vi "Send Packets.vi"(8 "error in (no error)":errorcluster, 9 "Delay before packets, sec":dbl=0.1 format="%#_13g", 10 "SG Power, dBm":dbl, 11 "IVI Refnum in":refnum<k15>) -> (0 "error out":errorcluster, 3 "IVI Refnum out":refnum<k15>)   [LabVIEW 2025, in "Nordic nRF52 DK DTM Test.lvlib"]
uses:
  Nordic nRF52 DK DTM Test.lvlib
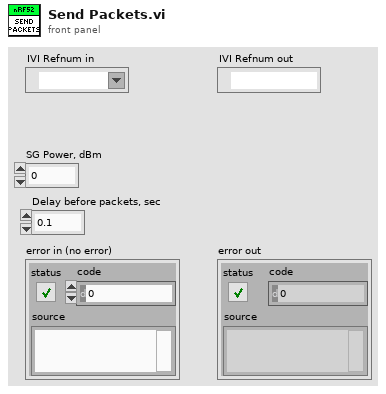
[diagram p1: front panel]
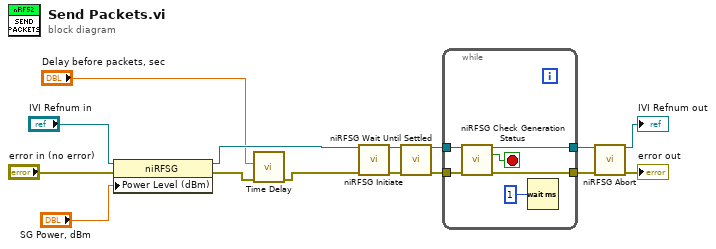
[diagram p0: block diagram]
diagram:
  n1 = property class="niRFSG"(reference="IVI Refnum in", error in="error in (no error)", "Power Level (dBm)"="SG Power, dBm") -> (reference out=w2:refnum<k15>, error out=w4:errorcluster)
  n2 = call "Time Delay"("error in (no error)"=w4, "Delay Time (s)"="Delay before packets, sec") -> ("error out"=w3:errorcluster)  [unwired: 9 in]
  n3 = call <instrlib>:"niRFSG Initiate.vi"("instrument handle"=w2, "error in"=w3) -> ("instrument handle out"=w9:refnum<k15>, "error out"=w10:errorcluster)  [unwired: 12 out]
  n4 = call <instrlib>:"niRFSG Wait Until Settled.vi"("instrument handle"=w9, "error in"=w10) -> ("instrument handle out"=w15:refnum<k15>, "error out"=w14:errorcluster)  [unwired: 12 in]
  n5 = while {
    tunnel: w14 -> [w21]
    tunnel: w15 -> [w19]
    tunnel: [w18] -> w7
    tunnel: [w17] -> w8
    stop <- w20 stop-if-true
    n6 = call <instrlib>:"niRFSG Check Generation Status.vi"("instrument handle"=w19, "error in"=w21) -> ("instrument handle out"=w18:refnum<k15>, "done?"=w20:bool, "error out"=w17:errorcluster)  [unwired: 11 in]
    n7 = Wait (ms)(milliseconds to wait=u32 1) -> ()  [unwired: 1 out]
  }
  n8 = call <instrlib>:"niRFSG Abort.vi"("instrument handle"=w7, "error in"=w8) -> ("instrument handle out"=→"IVI Refnum out":refnum<k15>, "error out"=→"error out":errorcluster)  [unwired: 12 in]
